vi "MAIN_merFISH_initialization.vi"(0 "queue DAQ":refnum<queue>, 1 "queue ASI stage":refnum<queue>, 2 "Measure QPD":bool caption="Calibration", 4 "queue CAMERA":refnum<queue>, 5 "VISA stage port":refnum<visa-resource-name>, 6 "queue FPGA":refnum<queue>, 7 "error in":errorcluster, 8 "queue valve":refnum<queue>, 9 "queue pump":refnum<queue>, 10 "Initialization status":T1, 11 "queue piezo":refnum<queue>, 12 "Exp time (s)":sgl, 15 "VISA resource Valve":refnum<visa-resource-name>, 17 "Autofocus lost Refnum":refnum<vi>) -> (19 "error out":errorcluster)   [LabVIEW 2015]
uses:
  CONTROLS/Q_camera_element.ctl
  CONTROLS/Q_ASI_stage_element.ctl
  CONTROLS/Q_DAQ_element.ctl
  CONTROLS/Q_MCL_piezo_element.ctl
  CONTROLS/Q_PUMP_element.ctl
  CONTROLS/Q_VALVE_element.ctl
  CONTROLS/Q_FPGA_element.ctl
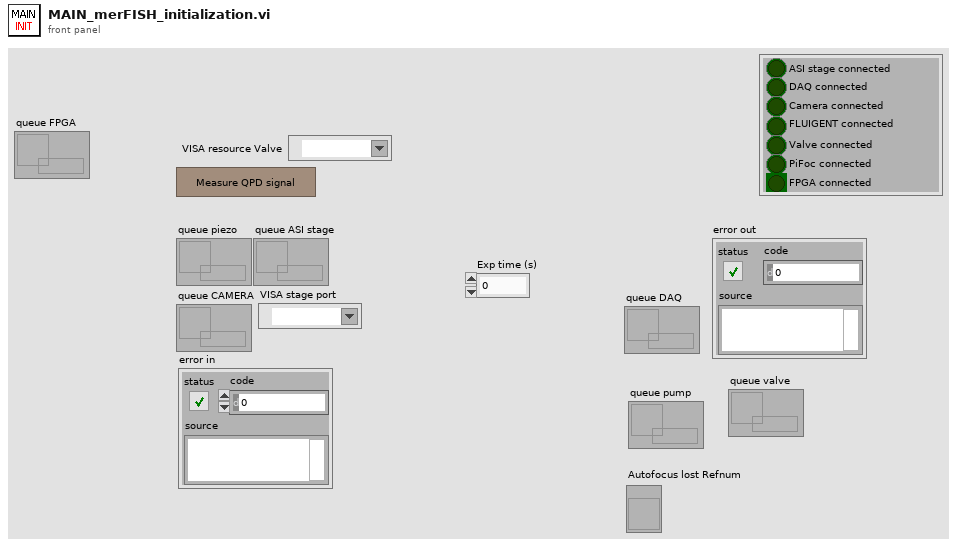
[diagram p1: front panel]
types:
  T1 = cluster{"ASI":bool, "DAQ":bool, "Camera":bool, "Pump":bool, "Valve":bool, "PiFoc":bool, "FPGA":bool}
  T2 = typedef "Q_ASI_stage_element.ctl" = cluster{"variant":variant, "Instruction":enum16{"ASI_idle", "ASI_initialize", "ASI_error", "ASI_security_stop", "ASI_read_XYZ", "ASI_up", "ASI_down", "ASI_left", "ASI_right", "ASI_save_XY", "ASI_move_to_XY", "ASI_brightfield", "ASI_init_scan", "ASI_init_merFISH", "ASI_move_to_XY_merFISH", "ASI_move_to_Z_merFISH", "ASI_init_autofocus_search_merFISH", "ASI_close_autofocus_search_merFISH", "ASI_adjust_piezo_autofocus_merFISH", "ASI_set_piezo_autofocus_to_reference_position_merFISH_TL", "ASI_close_merFISH", "ASI_stop"}}
  T3 = typedef "Q_DAQ_element.ctl" = cluster{"variant":variant, "Instruction":enum16{"DAQ_idle", "DAQ_initialize", "DAQ_error", "DAQ_security_stop", "DAQ_init_single_scan", "DAQ_single_scan", "DAQ_init_merFISH", "DAQ_scan_merFISH", "DAQ_photobleaching_merFISH", "DAQ_close_merFISH", "DAQ_stop"}}
  T4 = typedef "Q_MCL_piezo_element.ctl" = cluster{"variant":variant, "Instruction":enum16{"Piezo_idle", "Piezo_initialize", "Piezo_error", "Piezo_security_stop", "Piezo_read_z", "Piezo_move_z", "Piezo_keyboard_move", "Piezo_close_autofocus_calibration_ramp", "Piezo_change_init_state", "Piezo_init_autofocus", "Piezo_init_autofocus_merFISH_TL", "Piezo_autofocus", "Piezo_autofocus_merFISH_TL", "Piezo_stop_autofocus", "Piezo_stop_autofocus_merFISH_TL", "Piezo_autofocus_lost", "Piezo_resume_autofocus_merFISH_TL", "Piezo_check_z_position_merFISH_TL", "Piezo_init_ramp", "Piezo_move_z_ramp", "Piezo_close_ramp", "Piezo_close_merFISH", "Piezo_stop"}}
  T5 = typedef "Q_camera_element.ctl" = cluster{"variant":variant, "Instruction":enum16{"CAMERA_idle", "CAMERA_initialize", "CAMERA_error", "CAMERA_security_stop", "CAMERA_not_acquiring", "CAMERA_acquiring", "CAMERA_start_acquiring", "CAMERA_stop_acquiring", "CAMERA_change_exposure", "CAMERA_define_ROI", "CAMERA_cooler", "CAMERA_acquire_movie", "CAMERA_init_scan", "CAMERA_check_image_scan", "CAMERA_close_scan", "CAMERA_init_merFISH", "CAMERA_start_acquiring_merFISH", "CAMERA_close_scan_merFISH", "CAMERA_close_merFISH", "CAMERA_STOP"}}
  T6 = typedef "Q_PUMP_element.ctl" = cluster{"variant":variant, "Instruction":enum16{"PUMP_idle", "PUMP_initialize", "PUMP_error", "PUMP_security_stop", "PUMP_read_pressure", "PUMP_change_pressure", "PUMP_init_merFISH", "PUMP_change_presure_merFISH", "PUMP_zero_pressure_merFISH", "PUMP_close_merFISH", "PUMP_stop"}}
  T7 = typedef "Q_VALVE_element.ctl" = cluster{"variant":variant, "Instruction":enum16{"VALVE_idle", "VALVE_initialize", "VALVE_error", "VALVE_security_stop", "VALVE_change_position", "VALVE_two_way_valves", "VALVE_init_merFISH", "VALVE_stop"}}
  T8 = typedef "Q_FPGA_element.ctl" = cluster{"variant":variant, "Instruction":enum16{"FPGA_idle", "FPGA_initialize", "FPGA_error", "FPGA_security_stop", "FPGA_laser", "FPGA_start_stop_measure_QPD", "FPGA_measure_QPD", "FPGA_measure_QPD_noise", "FPGA_stop_measure_QPD", "FPGA_init_autofocus", "FPGA_init_single_scan", "FPGA_stop_single_scan", "FPGA_init_merFISH", "FPGA_measure_QPD_merFISH", "FPGA_init_scan_merFISH", "FPGA_scan_merFISH", "FPGA_close_merFISH", "FPGA_stop"}}
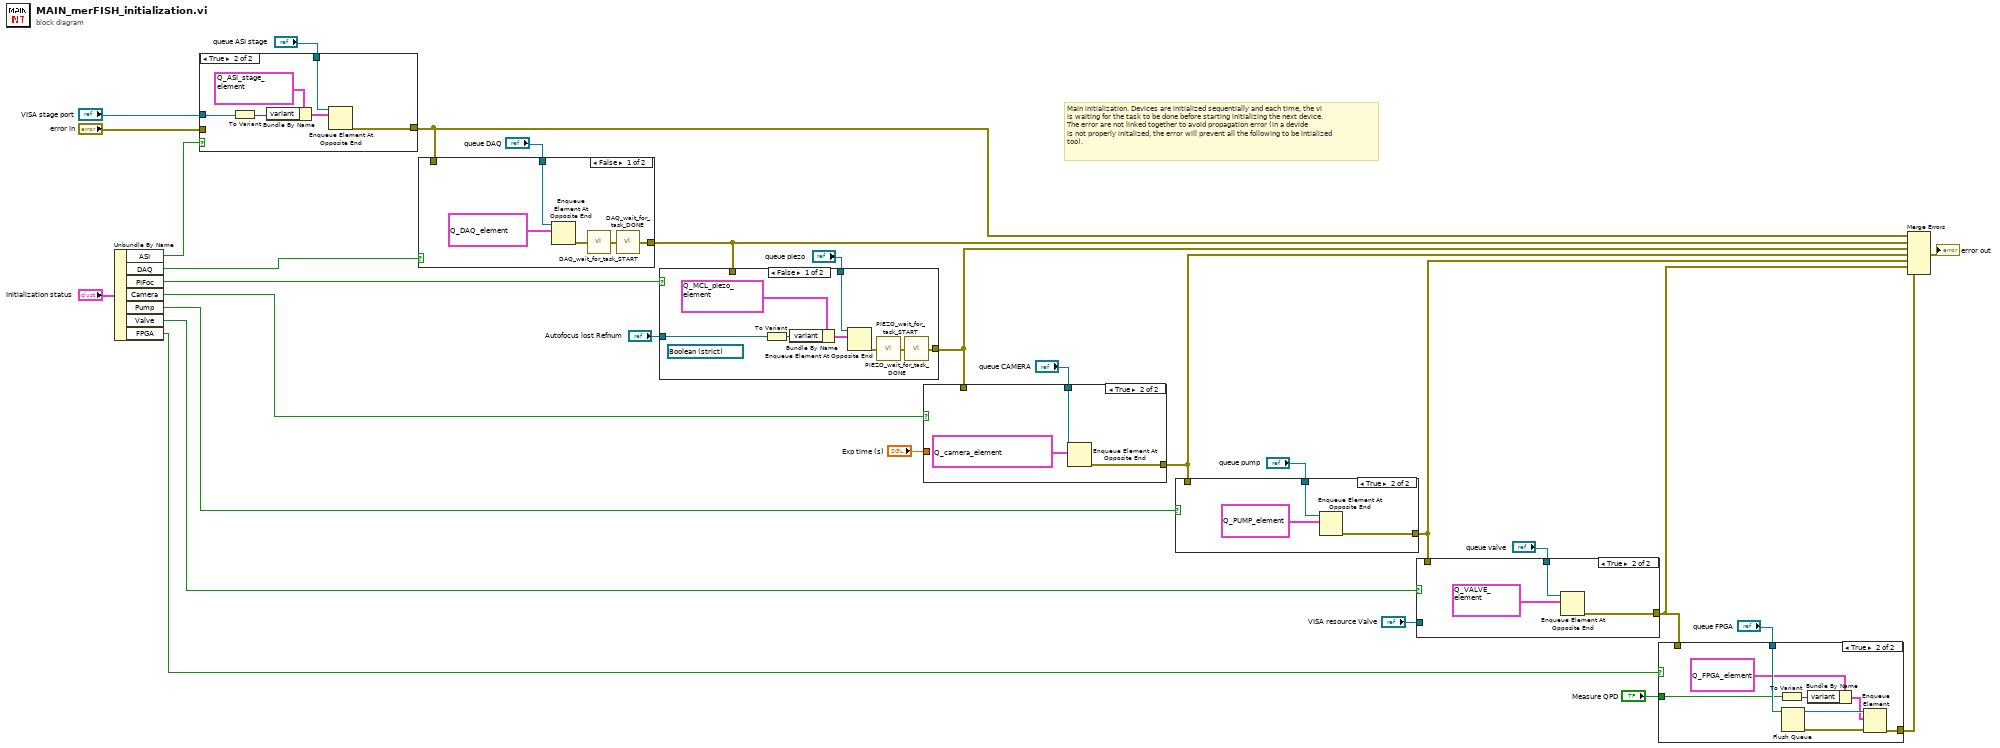
[diagram p0: block diagram]
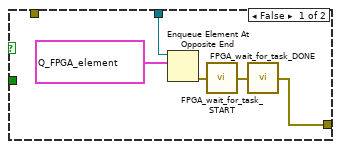
[diagram p2: hidden frame]
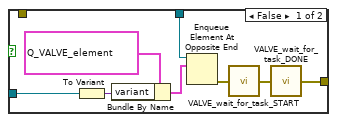
[diagram p3: hidden frame]
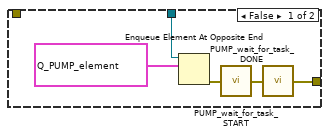
[diagram p4: hidden frame]
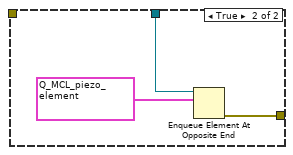
[diagram p5: hidden frame]
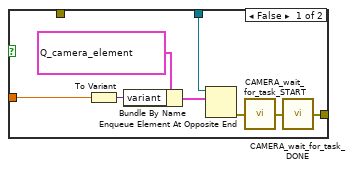
[diagram p6: hidden frame]
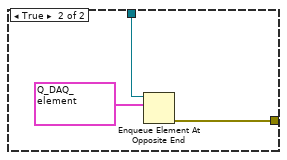
[diagram p7: hidden frame]
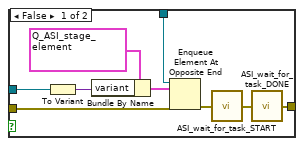
[diagram p8: hidden frame]
diagram:
  # "Main initialization. Devices are initialized sequentially and each time, the vi\nis waiting for the task to be done before starting initializing the next device.\nThe error are not linked together to avoid propagation error (in a devide\nis not properly initalized, the error will prevent all the following to be intialized\ntoo)."
  n1 = Unbundle By Name("Initialization status") -> ("ASI"=w27:bool, "DAQ"=w26:bool, "PiFoc"=w22:bool, "Camera"=w23:bool, "Pump"=w19:bool, "Valve"=w16:bool, "FPGA"=w3:bool)
  n2 = case shown="True" w27 {
    tunnel: [w31 w39] -> w15
    tunnel: "queue ASI stage" -> [w37 w44]
    tunnel: "VISA stage port" -> [w33 w40]
    tunnel: "error in" -> [w30 _]
    frame False {
      n3 = To Variant(anything=w33) -> (Variant=w34:variant)
      n4 = Bundle By Name(cluster=T2 {"variant"=variant, "Instruction"=enum."ASI_initialize"} ("Q_ASI_stage"), "variant"=w34) -> (w35:T2)
      n5 = Enqueue Element At Opposite End(queue=w37, element=w35, error in (no error)=w30) -> (error out=w38:errorcluster)  [unwired: 1 in, 2 out]
      n6 = call "ASI_wait_for_task_START.vi"("error in"=w38) -> ("error out"=w32:errorcluster)
      n7 = call "ASI_wait_for_task_DONE.vi"("error in"=w32) -> ("error out"=w31:errorcluster)
    }
    frame True {
      n8 = To Variant(anything=w40) -> (Variant=w41:variant)
      n9 = Bundle By Name(cluster=T2 {"variant"=variant, "Instruction"=enum."ASI_read_XYZ"} ("Q_ASI_stage"), "variant"=w41) -> (w42:T2)
      n10 = Enqueue Element At Opposite End(queue=w44, element=w42) -> (error out=w39:errorcluster)  [unwired: 2 in, 2 out]
    }
  }
  n11 = case shown="False" w26 {
    tunnel: "queue DAQ" -> [w49 w52]
    tunnel: [w47 w51] -> w14
    tunnel: w15 -> [_ _]
    frame False {
      n12 = Enqueue Element At Opposite End(queue=w49, element=T3 {"variant"=variant, "Instruction"=enum."DAQ_initialize"} ("Q_DAQ")) -> (error out=w46:errorcluster)  [unwired: 2 in, 2 out]
      n13 = call "DAQ_wait_for_task_START.vi"("error in"=w46) -> ("error out"=w48:errorcluster)
      n14 = call "DAQ_wait_for_task_DONE.vi"("error in"=w48) -> ("error out"=w47:errorcluster)
    }
    frame True {
      n15 = Enqueue Element At Opposite End(queue=w52, element=T3 {"variant"=variant, "Instruction"=enum."DAQ_idle"} ("Q_DAQ")) -> (error out=w51:errorcluster)  [unwired: 2 in, 2 out]
    }
  }
  n16 = case shown="False" w22 {
    tunnel: "queue piezo" -> [w57 w63]
    tunnel: [w58 w61] -> w13
    tunnel: w14 -> [_ _]
    tunnel: "Autofocus lost Refnum" -> [w53 _]
    frame False {
      (unwired) refnum<vi> refnum ("Autofocus lost Refnum")
      n17 = To Variant(anything=w53) -> (Variant=w55:variant)
      n18 = Bundle By Name(cluster=T4 {"variant"=variant, "Instruction"=enum."Piezo_initialize"} ("Q_MCL_Piezo"), "variant"=w55) -> (w56:T4)
      n19 = Enqueue Element At Opposite End(queue=w57, element=w56) -> (error out=w60:errorcluster)  [unwired: 2 in, 2 out]
      n20 = call "PIEZO_wait_for_task_START.vi"("error in"=w60) -> ("error out"=w59:errorcluster)
      n21 = call "PIEZO_wait_for_task_DONE.vi"("error in"=w59) -> ("error out"=w58:errorcluster)
    }
    frame True {
      n22 = Enqueue Element At Opposite End(queue=w63, element=T4 {"variant"=variant, "Instruction"=enum."Piezo_read_z"} ("Q_MCL_Piezo")) -> (error out=w61:errorcluster)  [unwired: 2 in, 2 out]
    }
  }
  n23 = case shown="True" w23 {
    tunnel: [w66 w72] -> w12
    tunnel: "queue CAMERA" -> [w65 w74]
    tunnel: "Exp time (s)" -> [w64 _]
    tunnel: w13 -> [_ _]
    frame False {
      n24 = To Variant(anything=w64) -> (Variant=w71:variant)
      n25 = Bundle By Name(cluster=T5 {"variant"=variant, "Instruction"=enum."CAMERA_initialize"} ("Q_ANDOR_element"), "variant"=w71) -> (w70:T5)
      n26 = Enqueue Element At Opposite End(queue=w65, element=w70) -> (error out=w68:errorcluster)  [unwired: 2 in, 2 out]
      n27 = call "CAMERA_wait_for_task_START.vi"("error in"=w68) -> ("error out"=w67:errorcluster)
      n28 = call "CAMERA_wait_for_task_DONE.vi"("error in"=w67) -> ("error out"=w66:errorcluster)
    }
    frame True {
      n29 = Enqueue Element At Opposite End(queue=w74, element=T5 {"variant"=variant, "Instruction"=enum."CAMERA_not_acquiring"} ("Q_ANDOR_element")) -> (error out=w72:errorcluster)  [unwired: 2 in, 2 out]
    }
  }
  n30 = case shown="True" w19 {
    tunnel: [w77 w81] -> w11
    tunnel: "queue pump" -> [w76 w82]
    tunnel: w12 -> [_ _]
    frame False {
      n31 = Enqueue Element At Opposite End(queue=w76, element=T6 {"variant"=variant, "Instruction"=enum."PUMP_initialize"} ("Q_PUMP")) -> (error out=w79:errorcluster)  [unwired: 2 in, 2 out]
      n32 = call "PUMP_wait_for_task_START.vi"("error in"=w79) -> ("error out"=w78:errorcluster)
      n33 = call "PUMP_wait_for_task_DONE.vi"("error in"=w78) -> ("error out"=w77:errorcluster)
    }
    frame True {
      n34 = Enqueue Element At Opposite End(queue=w82, element=T6 {"variant"=variant, "Instruction"=enum."PUMP_idle"} ("Q_PUMP")) -> (error out=w81:errorcluster)  [unwired: 2 in, 2 out]
    }
  }
  n35 = case shown="True" w16 {
    tunnel: [w88 w92] -> w4
    tunnel: "queue valve" -> [w87 w93]
    tunnel: w11 -> [_ _]
    tunnel: "VISA resource Valve" -> [w84 _]
    frame False {
      n36 = To Variant(anything=w84) -> (Variant=w86:variant)
      n37 = Bundle By Name(cluster=T7 {"variant"=variant, "Instruction"=enum."VALVE_initialize"} ("Q_VALVE"), "variant"=w86) -> (w83:T7)
      n38 = Enqueue Element At Opposite End(queue=w87, element=w83) -> (error out=w90:errorcluster)  [unwired: 2 in, 2 out]
      n39 = call "VALVE_wait_for_task_START.vi"("error in"=w90) -> ("error out"=w89:errorcluster)
      n40 = call "VALVE_wait_for_task_DONE.vi"("error in"=w89) -> ("error out"=w88:errorcluster)
    }
    frame True {
      n41 = Enqueue Element At Opposite End(queue=w93, element=T7 {"variant"=variant, "Instruction"=enum."VALVE_idle"} ("Q_VALVE")) -> (error out=w92:errorcluster)  [unwired: 2 in, 2 out]
    }
  }
  n42 = case shown="True" w3 {
    tunnel: [w97 w103] -> w5
    tunnel: "queue FPGA" -> [w95 w106]
    tunnel: w4 -> [_ _]
    tunnel: "Measure QPD" -> [_ w100]
    frame False {
      n43 = Enqueue Element At Opposite End(queue=w95, element=T8 {"variant"=variant, "Instruction"=enum."FPGA_initialize"}) -> (error out=w96:errorcluster)  [unwired: 2 in, 2 out]
      n44 = call "FPGA_wait_for_task_START.vi"("error in"=w96) -> ("error out"=w98:errorcluster)
      n45 = call "FPGA_wait_for_task_DONE.vi"("error in"=w98) -> ("error out"=w97:errorcluster)
    }
    frame True {
      n46 = To Variant(anything=w100) -> (Variant=w99:variant)
      n47 = Flush Queue(queue=w106) -> (queue out=w104:refnum<queue>, error out=w105:errorcluster)  [unwired: 1 in, 1 out]
      n48 = Bundle By Name(cluster=T8 {"variant"=variant, "Instruction"=enum."FPGA_idle"} ("element"), "variant"=w99) -> (w101:T8)
      n49 = Enqueue Element(queue=w104, element=w101, error in (no error)=w105) -> (error out=w103:errorcluster)  [unwired: 1 in, 2 out]
    }
  }
  n50 = Merge Errors(w15, w14, w13, w12, w11, w4, w5) -> (→"error out":errorcluster)
